vi "Get Window Handle.vi"(4 "error in (no error)":errorcluster, 6 "parentwindow handle (NULL)":u32, 7 "window name (\"\")":string) -> (0 "error out":errorcluster, 3 "hWnd":u32)   [LabVIEW 2014]
doc: "This VI will use the FindWindow API function to retrieve a window refnum for the window identified by window name. 'window name' is the text appearing in the title bar of a window. If the window cannot be found, the window refnum out will be 'Not a Window Refnum', and an error will occur."
uses:
  USER32.DLL
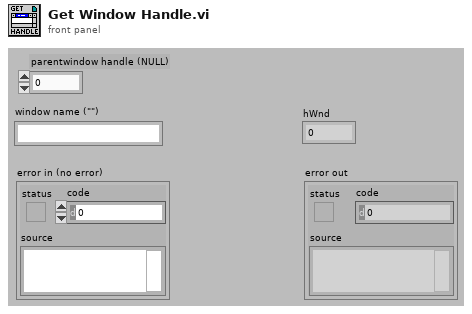
[diagram p1: front panel]
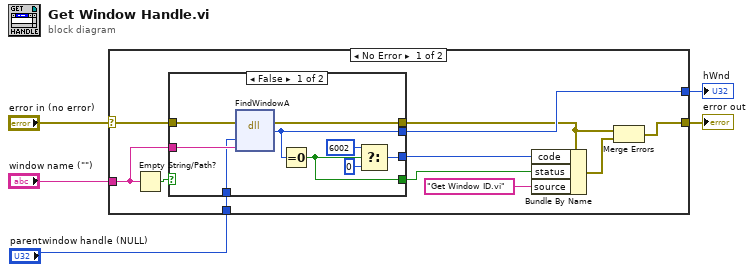
[diagram p0: block diagram]
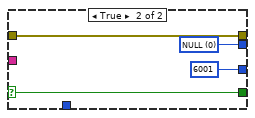
[diagram p2: hidden frame]
diagram:
  n1 = case shown="No Error" "error in (no error)" {
    selector: "error in (no error)" -> [w8 w30]
    tunnel: [w10 w30] -> w3
    tunnel: [w13 _] -> w2
    tunnel: "window name (\"\")" -> [w9 _]
    tunnel: "parentwindow handle (NULL)" -> [w6 _]
    frame No Error {
      n2 = Empty String/Path?(string/path=w9) -> (empty?=w12:bool)
      n3 = case shown="False" w12 {
        selector: w12 -> [_ w27]
        tunnel: [w25 w28] -> w13
        tunnel: [w24 w27] -> w15
        tunnel: [w23 6001] -> w16
        tunnel: w9 -> [w20 _]
        tunnel: w8 -> [w19 w26]
        tunnel: [w18 w26] -> w7
        tunnel: w6 -> [w17 _]
        frame False {
          n4 = dll-call lib="user32.dll" fn="FindWindowA" label="FindWindow"(error in=w19, "lpszClassName"=w17, "lpszWindowName"=w20) -> (error out=w18:errorcluster, "hWnd"=w25:u32)  [unwired: 4 in, 1 out]
          n5 = Equal To 0?(x=w25) -> (x = 0?=w24:bool)
          n6 = Select(t=6002, s=w24, f=0) -> (s? t:f=w23:i32)
        }
        frame True {
          w28 = u16 0 items=["NULL"]
        }
      }
      n7 = Bundle By Name(cluster=w7, "code"=w16, "status"=w15, "source"="Get Window ID.vi") -> (w11:errorcluster)
      n8 = Merge Errors(w7, w11) -> (w10:errorcluster)
    }
    frame Error {
    }
  }
  "error out" <- w3
  "hWnd" <- w2
